vi "Analog DC Signal.vi"(1 "dt":dbl, 2 "Amplitude":dbl) -> (0 "DC Analog Signal":waveform(dbl)(graph))   [LabVIEW 2019, in "SubVIs.lvlib" / "Torque VI.lvlib"]
uses:
  Torque VI.lvlib
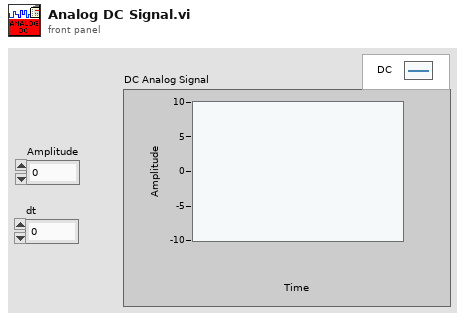
[diagram p1: front panel]
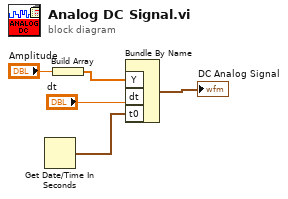
[diagram p0: block diagram]
diagram:
  n1 = Get Date/Time In Seconds() -> (seconds since 1Jan1904=w4:timestamp)
  n2 = Build Array "Build Array"("Amplitude") -> (w2:dbl[])
  n3 = Bundle By Name("Y"=w2, "dt"="dt", "t0"=w4) -> (→"DC Analog Signal":waveform(dbl))  [unwired: 1 in]
